vi "Server.vi"() -> ()   [LabVIEW 2016]
uses:
  <vilib>/rvi/eio/common/nirviEmuClasses.ctl
  <vilib>/rvi/Emulation/niFpgaSctlEmulationGetInTimedLoop.vi
  <vilib>/rvi/Emulation/niFpgaProcessEmulError.vi
  <vilib>/rvi/eio/common/nirviEmuTemplateMethod_errors.vi
  <vilib>/rvi/Emulation/niFpgaEmulationIsFPGAContextNoSignature.vi
  <vilib>/rvi/DataTransferAndStorage/Container/Common/niFpgaContainerGetUniqueNameForEmu.vi
  <vilib>/rvi/Memory/Memory_Emulation/niFpgaMemoryEmulationCacheClearOnFirstRun.vi
  <vilib>/rvi/Memory/Memory_Emulation/nirvimemoryEmulationManagerCache_MakeExclusive.vi
  <vilib>/rvi/Memory/Memory_Emulation/niFpgaMemoryEmulationValidateCache.vi
  <vilib>/rvi/Memory/Memory_Emulation/nirvimemoryEmulationManagerCache_InsertValue.vi
  <vilib>/Utility/error.llb/Clear Errors.vi
  <vilib>/rvi/Memory/Memory_Emulation/nirvimemoryEmulationManagerCache_ReleaseExclusive.vi
  <vilib>/rvi/Memory/Memory_Emulation/nirvimemoryEmulationManagerCache_GetValue.vi
  <vilib>/rvi/Memory/Memory_Emulation/nirvimemoryEmulationManagerCache_SetValue.vi
  <vilib>/rvi/Emulation/niFpgaGetClockAttributes.vi
  <vilib>/rvi/Emulation/niFpgaEmulationReportErrorSimple.vi
  <vilib>/rvi/Emulation/niFpgaCriticalErrorInLSC.vi
  <vilib>/rvi/eio/common/nirviEmuTemplateMethod_noerrors.vi
  <vilib>/rvi/errors/niFpgaSetErrorForExecOnDevCompSimple.vi
  <vilib>/rvi/eio/common/nirviEmuReportErrorAndStop.vi
  <vilib>/rvi/FIFO/Fifo_Resource/nirvififoEmulationSetSize.vi
  <vilib>/rvi/FIFO/Fifo_Resource/nirviFifoEmulationQueueMgr.vi
  <instcachedir>/0/nirviFifoEmulationQueueMgr_E5CAEC123FF24DC58D834DCA3CDAA9B5.lvgen/nirviFifoEmulationQueueMgr_E5CAEC123FF24DC58D834DCA3CDAA9B5_001.vi
  <vilib>/rvi/FIFO/Fifo_Resource/nirvififoEmulationCreateLock.vi
  <vilib>/rvi/FIFO/Fifo_Resource/nirvififoEmulationObtainLock.vi
  <vilib>/rvi/FIFO/Fifo_Resource/nirvififoEmulationReleaseLock.vi
  <vilib>/rvi/occurrence/nirviWaitOnOccurrenceBase.vi
  <vilib>/rvi/errors/nirviReportUnexpectedCaseInternalError.vi
  <vilib>/rvi/errors/nirviReportUnexpectedCaseInternalError (U32).vi
  <vilib>/rvi/FIFO/Fifo_Resource/nirvififoEmulationDetermineInputValidOut.vi
  <vilib>/eio/EIOGrowableMethodNode/genericMethod/EIOGrowableMethodNode.xnode
  <vilib>/rvi/eio/nirviEIOMethodImplementation/nirviEIOMethodImplementation.xnode
  <vilib>/rvi/eio/nirviErrorMerge/nirviErrorMerge.xnode
  <vilib>/rvi/DataTransferAndStorage/Container/XNode/niFpgaContainer.xnode
  <vilib>/rvi/DataTransferAndStorage/Register/Emulation/niFpgaRegisterEmulation.vi
  <vilib>/eio/EIONode/EIONode.xnode
  <vilib>/rvi/FIFO/Fifo_Resource/nirvififoEmulationRead.vi
  <vilib>/rvi/FIFO/Fifo_Resource/nirvififoEmulationWrite.vi
panel:
  out "Samp2Collect":i32
  out "IO State":T1(ring)
  out "Attempts to Transmit":u64
  out "Timed Out":bool
  out "Transmit Out":bool
  out "CRD Data Loop":bool
  out "Temperatures":T2
  out "Sensor Status":u8
  in  "PAS Laser 1 Enable":bool
  in  "PAS Laser 2 Enable":bool
  in  "CRD Laser Enable":bool
  in  "f1":u32
  in  "f0":u32
  in  "PAS Speaker Enable":bool
  in  "O2 Add":bool
  in  "uv light enable":bool
  in  "O3 Add":bool
  in  "Filter Ctl":bool
  in  "Transmit?":bool
  in  "CRDSampData":u32
  in  "Speaker":cluster{"Vscale":fxp<+,32,0>, "Offset":i16}
  in  "Stop":bool
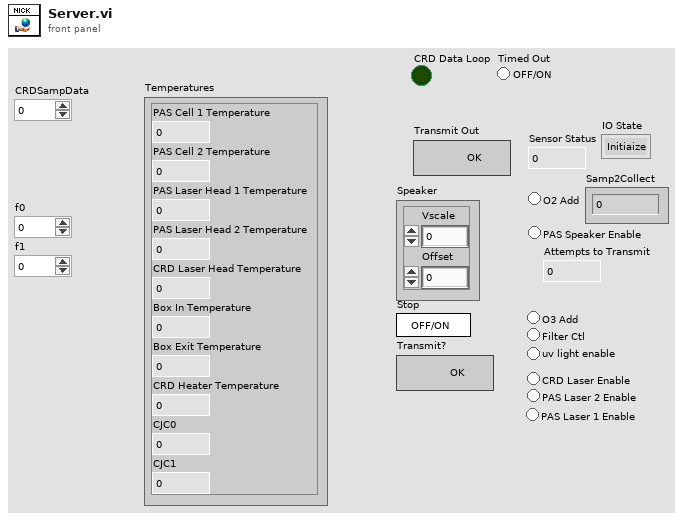
[diagram p1: front panel]
types:
  T1 = enum16{"Initiaize", "Running", "Stopped", "NOOP"}
  T2 = cluster{"PAS Cell 1 Temperature":fxp<+/-,24,-2>, "PAS Cell 2 Temperature":fxp<+/-,24,-2>, "PAS Laser Head 1 Temperature":fxp<+/-,24,-2>, "PAS Laser Head 2 Temperature":fxp<+/-,24,-2>, "CRD Laser Head Temperature":fxp<+/-,24,-2>, "Box In Temperature":fxp<+/-,24,-2>, "Box Exit Temperature":fxp<+/-,24,-2>, "CRD Heater Temperature":fxp<+/-,24,-2>, "CJC0":fxp<+/-,24,-2>, "CJC1":fxp<+/-,24,-2>}
  T3 = typedef "nirviEmuClasses.ctl" = enum16{"IO Read", "IO Write", "Method", "Property Read", "Property Write"}
  T4 = cluster{"PAS Cell 1 Temperature":fxp<+/-,24,-2>, "PAS Cell 2 Temperature":fxp<+/-,24,-2>, "PAS Laser Head 1 Temperature":fxp<+/-,24,-2>, "PAS Laser Head 2 Temperature":fxp<+/-,24,-2>, "CRD Laser Head Temperature":fxp<+/-,24,-2>, "Box In Temperature":fxp<+/-,24,-2>, "Box Exit Temperature":fxp<+/-,24,-2>, "CRD Heater Temperature":fxp<+/-,24,-2>, "Mod5/CJC0":fxp<+/-,24,-2>, "Mod5/CJC1":fxp<+/-,24,-2>}
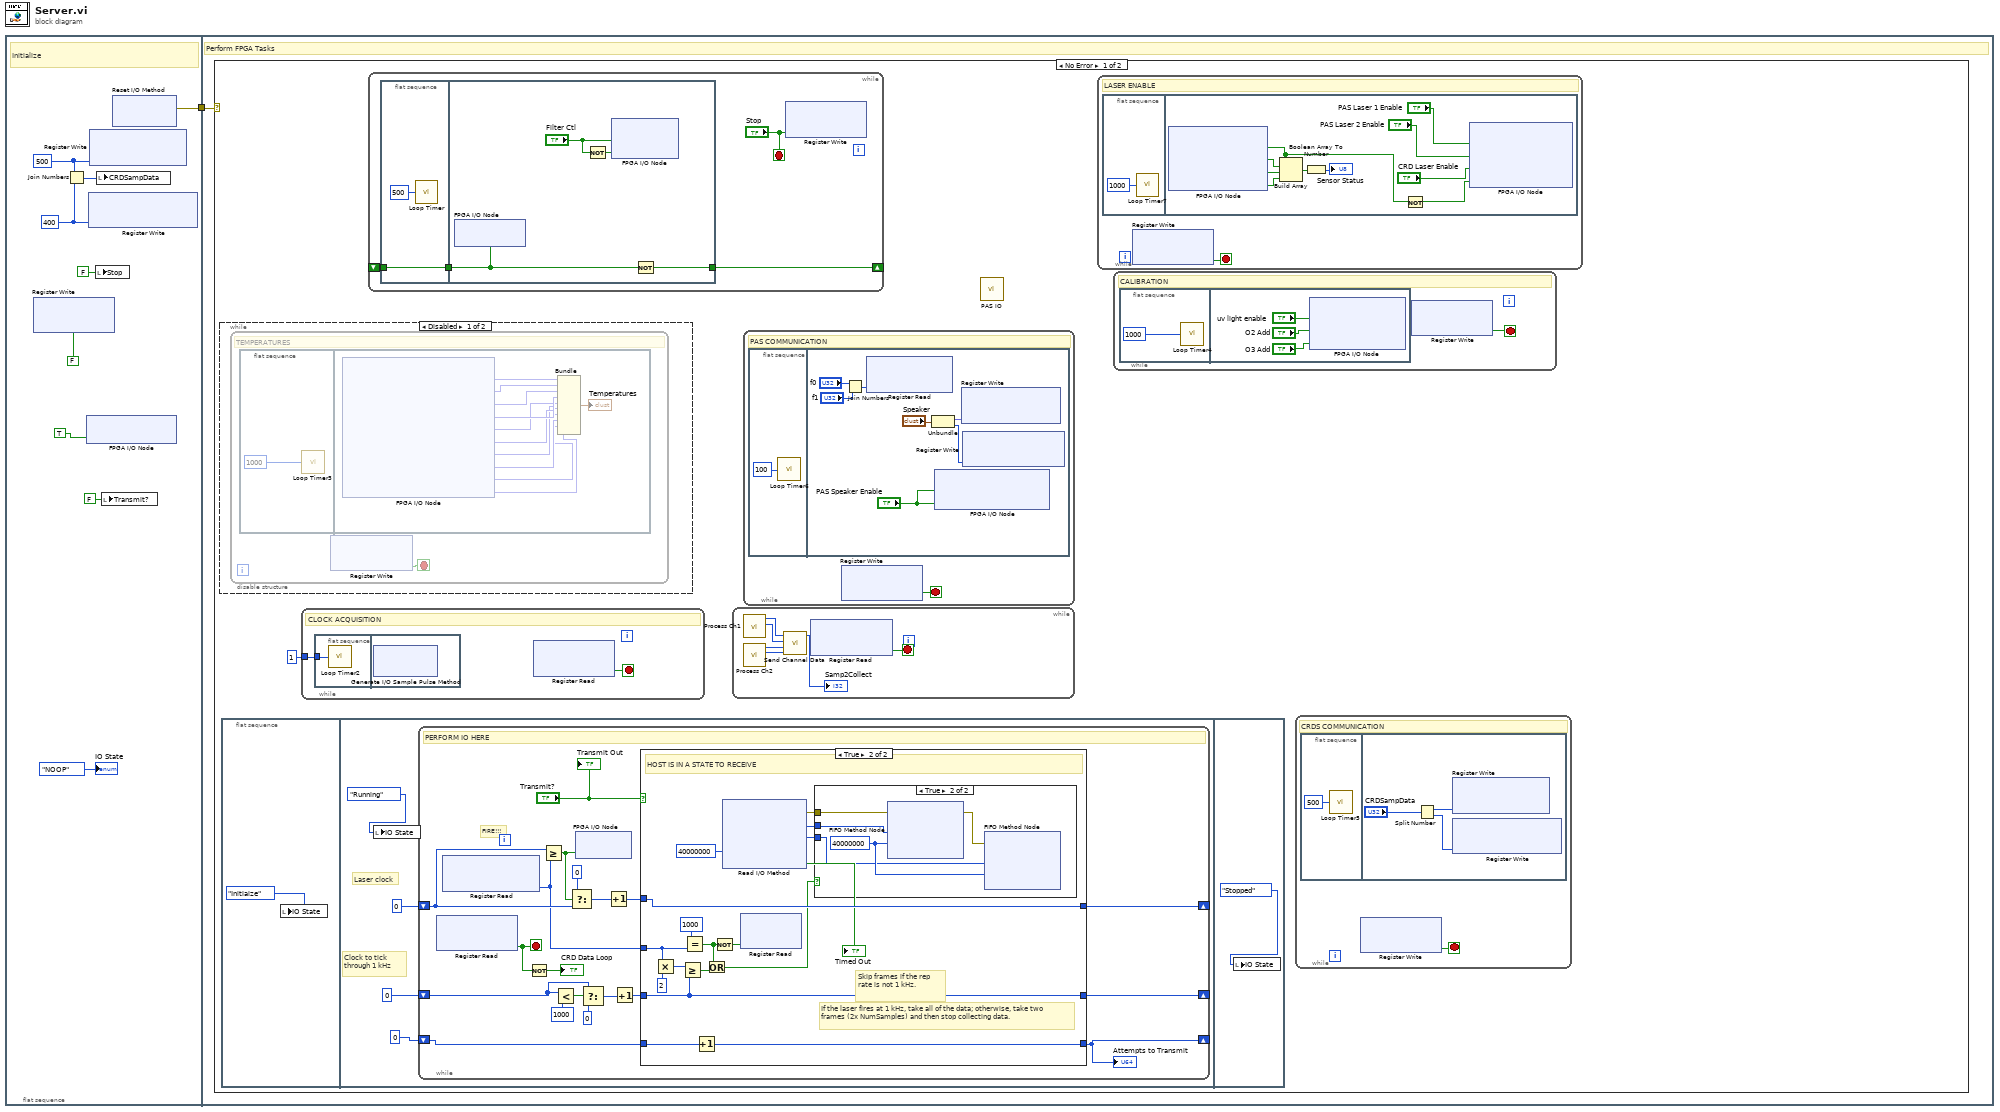
[diagram p0: block diagram]
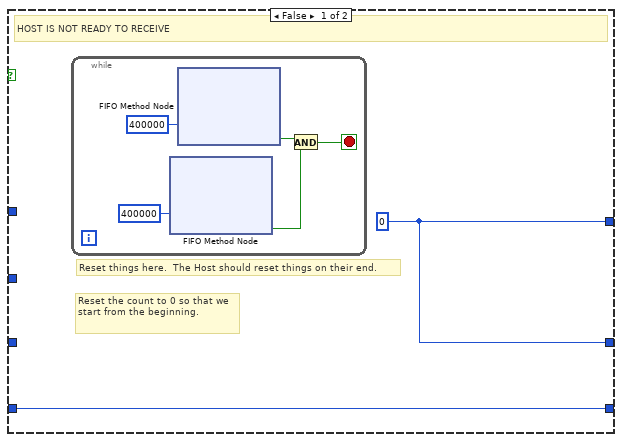
[diagram p3: hidden frame]
diagram:
  n1 = flat-sequence {
    tunnel: [w10] -> w1
    tunnel: w1 -> [w55]
    frame #0 {
      w7 = u16 500 ("Data")
      w6 = u16 400 ("Data")
      # "Initialize"
      n2 = xnode ("Register Write")("Data"=FALSE) -> ()  [unwired: 1 in, 1 out]
      n3 = Join Numbers(hi=w7, lo=w6) -> ((hi.lo)=w5:u32)
      n4 = xnode "FPGA I/O Node"("USB Hub Relay"=TRUE) -> ()  [unwired: 1 in, 1 out]
      n5 = xnode ("Register Write")("Data"=w6) -> ()  [unwired: 1 in, 1 out]
      n6 = xnode ("Register Write")("Data"=w7) -> ()  [unwired: 1 in, 1 out]
      n7 = local write "Stop"(FALSE ("Stop")) -> ()
      n8 = local write "CRDSampData"(w5) -> ()
      n9 = local write "Transmit?"(FALSE ("Transmit?")) -> ()
      n10 = xnode "Reset I/O Method"() -> ("error out"=w10:errorcluster)  [unwired: 2 in, 1 out]
      "IO State" <- T1."NOOP"
    }
    frame #1 {
      # "Perform FPGA Tasks"
      n11 = case shown="No Error" w55 {
        frame No Error {
          n12 = disable-structure shown="Disabled" {
            frame Disabled {
              n13 = while {
                stop <- w57 stop-if-true
                # "TEMPERATURES"
                n14 = flat-sequence {
                  frame #0 {
                    n15 = call "Loop Timer3"("Count(mSec)"=u32 1000 ("Sample Period (uSec)")) -> ()  [unwired: 1 out]
                  }
                  frame #1 {
                    n16 = xnode "FPGA I/O Node"() -> ("PAS Cell 1 Temperature"=w69:fxp<+/-,24,-2>, "PAS Cell 2 Temperature"=w68:fxp<+/-,24,-2>, "PAS Laser Head 1 Temperature"=w67:fxp<+/-,24,-2>, "PAS Laser Head 2 Temperature"=w66:fxp<+/-,24,-2>, "CRD Laser Head Temperature"=w65:fxp<+/-,24,-2>, "Box In Temperature"=w64:fxp<+/-,24,-2>, "Box Exit Temperature"=w63:fxp<+/-,24,-2>, "CRD Heater Temperature"=w62:fxp<+/-,24,-2>, "Mod5/CJC0"=w61:fxp<+/-,24,-2>, "Mod5/CJC1"=w60:fxp<+/-,24,-2>)  [unwired: 10 in, 10 out]
                    n17 = Bundle("PAS Cell 1 Temperature"=w69, "PAS Cell 2 Temperature"=w68, "PAS Laser Head 1 Temperature"=w67, "PAS Laser Head 2 Temperature"=w66, "CRD Laser Head Temperature"=w65, "Box In Temperature"=w64, "Box Exit Temperature"=w63, "CRD Heater Temperature"=w62, "Mod5/CJC0"=w61, "Mod5/CJC1"=w60) -> (→"Temperatures":T4)  [unwired: 1 in]
                  }
                }
                n18 = xnode ("Register Write")() -> ("Data"=w57:bool)  [unwired: 1 in, 1 out]
              }
            }
            frame Enabled {
            }
          }
          n19 = flat-sequence {
            frame #0 {
              n20 = local write "IO State"(T1."Initiaize") -> ()
            }
            frame #1 {
              # "Laser clock"
              # "Clock to tick through 1 kHz"
              n21 = local write "IO State"(T1."Running") -> ()
              n22 = while {
                shift-right: [w90] -> _
                shift-left: u16 0 ("Number of Samples") -> [w91]
                shift-right: [w82] -> _
                shift-left: u16 0 ("Number of Samples") -> [w80]
                shift-right: [w75] -> _
                shift-left: u64 0 ("Number of Samples") -> [w76]
                stop <- w78 stop-if-true
                # "FIRE!!!"
                # "PERFORM IO HERE"
                n23 = xnode ("Register Read")() -> ("Data"=w78:bool)  [unwired: 1 in, 1 out]
                n24 = xnode ("Register Read")() -> ("Data"=w85:u16)  [unwired: 1 in, 1 out]
                n25 = Not(x=w78) -> (.not. x?=→"CRD Data Loop":bool)
                n26 = Greater Or Equal?(x=w91, y=w85) -> (x >= y?=w92:bool)
                n27 = Less?(x=w80, y=u16 1000) -> (x < y?=w84:bool)
                n28 = Select(t=u16 0 ("Number of Samples"), s=w92, f=w91) -> (s? t:f=w89:u16)
                n29 = xnode "FPGA I/O Node"("CRDS"=w92) -> ()  [unwired: 1 in, 1 out]
                n30 = Select(t=w80, s=w84, f=u16 0 ("Number of Samples")) -> (s? t:f=w87:u16)
                n31 = Increment(x=w89) -> (x+1=w88:u16)
                n32 = Increment(x=w87) -> (x+1=w83:u16)
                n33 = case shown="True" "Transmit?" {
                  tunnel: w88 -> [_ w117]
                  tunnel: [w95 w117] -> w90
                  tunnel: w85 -> [_ w113]
                  tunnel: w83 -> [_ w108]
                  tunnel: [w95 w108] -> w82
                  tunnel: w76 -> [w94 w102]
                  tunnel: [w94 w101] -> w75
                  frame False {
                    w95 = u16 0 ("Number of Samples")
                    # "Reset things here.  The Host should reset things on their end."
                    # "Reset the count to 0 so that we start from the beginning."
                    # "HOST IS NOT READY TO RECEIVE"
                    n34 = while {
                      stop <- w96 stop-if-true
                      n35 = xnode ("FIFO Method Node")("Timeout"=400000) -> ("Timed Out?"=w97:bool)  [unwired: 1 in, 2 out]
                      n36 = xnode ("FIFO Method Node")("Timeout"=400000) -> ("Timed Out?"=w98:bool)  [unwired: 1 in, 2 out]
                      n37 = And(x=w98, y=w97) -> (x .and. y?=w96:bool)
                    }
                  }
                  frame True {
                    # "Skip frames if the rep rate is not 1 kHz."
                    # "If the laser fires at 1 kHz, take all of the data; otherwise, take two frames (2x NumSamples) and then stop collecting data."
                    # "HOST IS IN A STATE TO RECEIVE"
                    n38 = Multiply(x=w113, y=u16 2) -> (x*y=w111:u16)
                    n39 = Greater Or Equal?(x=w111, y=w108) -> (x >= y?=w110:bool)
                    n40 = Equal?(x=u16 1000, y=w113) -> (x = y?=w115:bool)
                    n41 = Increment(x=w102) -> (x+1=w101:u64)
                    n42 = Or(x=w115, y=w110) -> (x .or. y?=w109:bool)
                    n43 = Not(x=w115) -> (.not. x?=w114:bool)
                    n44 = xnode "Read I/O Method"("Timeout"=40000000) -> ("error out"=w105:errorcluster, "CRD Las Ch 1"=w106:i16, "CRD Las Ch 2"=w104:i16, "Timed Out"=→"Timed Out":bool)  [unwired: 3 in, 2 out]
                    n45 = xnode ("Register Read")("Data"=w114) -> ()  [unwired: 1 in, 1 out]
                    n46 = case shown="True" w109 {
                      tunnel: w106 -> [_ w230]
                      tunnel: w105 -> [_ w229]
                      tunnel: w104 -> [_ w227]
                      frame False {
                      }
                      frame True {
                        w228 = 40000000 ("Timeout")
                        n47 = xnode ("FIFO Method Node")("Element"=w230, "Timeout"=w228, "error in (no error)"=w229) -> ("error out"=w226:errorcluster)  [unwired: 1 in, 2 out]
                        n48 = xnode ("FIFO Method Node")("Element"=w227, "Timeout"=w228, "error in (no error)"=w226) -> ()  [unwired: 1 in, 3 out]
                      }
                    }
                  }
                }
                "Attempts to Transmit" <- w75
                "Transmit Out" <- "Transmit?"
              }
            }
            frame #2 {
              n49 = local write "IO State"(T1."Stopped") -> ()
            }
          }
          n50 = while {
            tunnel: u32 1 ("Sample Period (uSec)") -> [w251]
            stop <- w250 stop-if-true
            # "CLOCK ACQUISITION"
            n51 = flat-sequence {
              tunnel: w251 -> [w252]
              frame #0 {
                n52 = call "Loop Timer2"("Count(uSec)"=w252) -> ()  [unwired: 1 out]
              }
              frame #1 {
                n53 = xnode "Generate I/O Sample Pulse Method"() -> ()  [unwired: 2 in, 2 out]
              }
            }
            n54 = xnode ("Register Read")() -> ("Data"=w250:bool)  [unwired: 1 in, 1 out]
          }
          n55 = while {
            shift-right: [w281] -> _
            shift-left: _ -> [w280]
            stop <- "Stop" stop-if-true
            n56 = flat-sequence {
              tunnel: w280 -> [w283]
              tunnel: [w283] -> w278
              tunnel: [w287] -> w281
              tunnel: w278 -> [w286]
              frame #0 {
                n57 = call "Loop Timer"("Count(mSec)"=u32 500) -> ()  [unwired: 1 out]
              }
              frame #1 {
                n58 = xnode "FPGA I/O Node"("Heartbeat"=w286) -> ()  [unwired: 1 in, 1 out]
                n59 = Not(x="Filter Ctl") -> (.not. x?=w284:bool)
                n60 = xnode "FPGA I/O Node"("hb 1 ctl 1"="Filter Ctl", "hb 1 ctl 2"=w284) -> ()  [unwired: 2 in, 2 out]
                n61 = Not(x=w286) -> (.not. x?=w287:bool)
              }
            }
            n62 = xnode ("Register Write")("Data"="Stop") -> ()  [unwired: 1 in, 1 out]
          }
          n63 = while {
            stop <- w245 stop-if-true
            n64 = call "Process Ch1.vi"() -> ("Max1"=w248:u32, "Max0"=w249:u32)  [unwired: 10 in]
            n65 = call "Process Ch2.vi"() -> ("Max4"=w246:u32, "Max3"=w247:u32)  [unwired: 10 in]
            n66 = call "Send Channel Data.vi"("Max3"=w246, "Max2"=w247, "Max1"=w248, "Max0"=w249) -> ("32bit integer"=→"Samp2Collect":i32)  [unwired: 7 in]
            n67 = xnode ("Register Read")() -> ("Data"=w245:bool)  [unwired: 1 in, 1 out]
          }
          n68 = while {
            stop <- w259 stop-if-true
            # "PAS COMMUNICATION"
            n69 = flat-sequence {
              frame #0 {
                n70 = call "Loop Timer6"("Count(mSec)"=u32 100) -> ()  [unwired: 1 out]
              }
              frame #1 {
                n71 = Join Numbers(hi="f0", lo="f1") -> ((hi.lo)=w262:u64)
                n72 = xnode ("Register Read")("Data"=w262) -> ()  [unwired: 1 in, 1 out]
                n73 = Unbundle("Speaker") -> ("Vscale"=w267:fxp<+,32,0>, "Offset"=w266:i16)
                n74 = xnode "FPGA I/O Node"("PAS Speaker Enable 1"="PAS Speaker Enable", "PAS Speaker Enable 2"="PAS Speaker Enable") -> ()  [unwired: 2 in, 2 out]
                n75 = xnode ("Register Write")("Data"=w267) -> ()  [unwired: 1 in, 1 out]
                n76 = xnode ("Register Write")("Data"=w266) -> ()  [unwired: 1 in, 1 out]
              }
            }
            n77 = xnode ("Register Write")() -> ("Data"=w259:bool)  [unwired: 1 in, 1 out]
          }
          n78 = call "PAS IO.vi"() -> ()  [unwired: 20 in]
          n79 = while {
            stop <- w232 stop-if-true
            # "LASER ENABLE"
            n80 = flat-sequence {
              frame #0 {
                n81 = call "Loop Timer7"("Count(mSec)"=u32 1000) -> ()  [unwired: 1 out]
              }
              frame #1 {
                n82 = xnode "FPGA I/O Node"() -> ("Interlock Sense"=w235:bool, "hb 1 status 1"=w239:bool, "hb 1 status 2"=w238:bool, "Soft Power Down"=w237:bool)  [unwired: 4 in, 4 out]
                n83 = Build Array(w235, w239, w238, w237) -> (w236:bool[])
                n84 = Boolean Array To Number(Boolean array=w236) -> (number=→"Sensor Status":u8)
                n85 = Not(x=w235) -> (.not. x?=w234:bool)
                n86 = xnode "FPGA I/O Node"("PAS Laser Relay 1"="PAS Laser 1 Enable", "PAS Laser Relay 2"="PAS Laser 2 Enable", "CRD Laser Enable"="CRD Laser Enable", "Interlock Indicator"=w234) -> ()  [unwired: 4 in, 4 out]
              }
            }
            n87 = xnode ("Register Write")() -> ("Data"=w232:bool)  [unwired: 1 in, 1 out]
          }
          n88 = while {
            stop <- w273 stop-if-true
            # "CALIBRATION"
            n89 = flat-sequence {
              frame #0 {
                n90 = call "Loop Timer4"("Count(mSec)"=u32 1000 ("Sample Period (uSec)")) -> ()  [unwired: 1 out]
              }
              frame #1 {
                n91 = xnode "FPGA I/O Node"("uv light enable"="uv light enable", "Solenoid Relay 1"="O2 Add", "Solenoid Relay 2"="O3 Add") -> ()  [unwired: 3 in, 3 out]
              }
            }
            n92 = xnode ("Register Write")() -> ("Data"=w273:bool)  [unwired: 1 in, 1 out]
          }
          n93 = while {
            stop <- w268 stop-if-true
            # "CRDS COMMUNICATION"
            n94 = flat-sequence {
              frame #0 {
                n95 = call "Loop Timer5"("Count(mSec)"=u32 500) -> ()  [unwired: 1 out]
              }
              frame #1 {
                n96 = Split Number(x="CRDSampData") -> (hi(x)=w271:u16, lo(x)=w272:u16)
                n97 = xnode ("Register Write")("Data"=w271) -> ()  [unwired: 1 in, 1 out]
                n98 = xnode ("Register Write")("Data"=w272) -> ()  [unwired: 1 in, 1 out]
              }
            }
            n99 = xnode ("Register Write")() -> ("Data"=w268:bool)  [unwired: 1 in, 1 out]
          }
        }
        frame Error {
        }
      }
    }
  }
